vi "ArmR-L-EToXYZ.vi"(9 "Extend":dbl, 10 "Lift":dbl, 11 "Rotate":dbl) -> (1 "z":dbl, 2 "y":dbl, 3 "x":dbl)   [LabVIEW 2020]
uses:
  <vilib>/Rock Robotics/WPI/ThirdParty/JAS_Junk/TrajLib/Trajectory_Library.lvlib
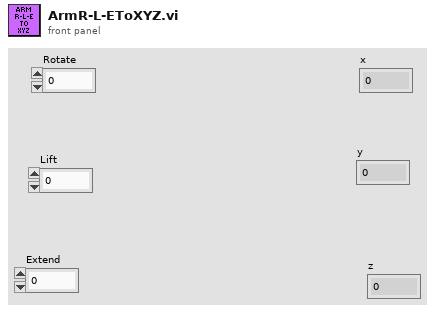
[diagram p1: front panel]
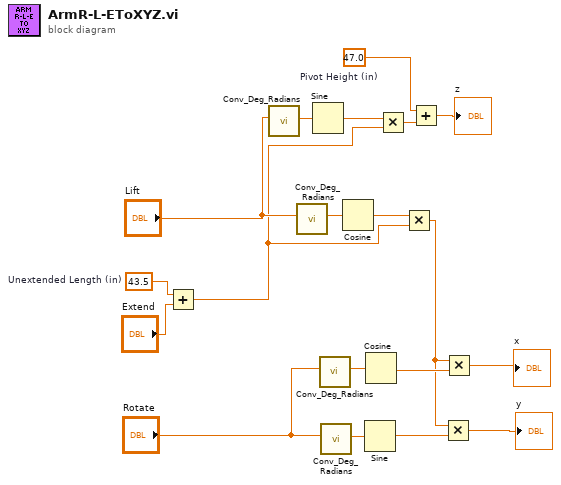
[diagram p0: block diagram]
diagram:
  w1 = 47.0  # Pivot Height (in)
  w18 = 43.5  # Unextended Length (in)
  n1 = Add(x=w18, y="Extend") -> (x+y=w12:dbl)
  n2 = call <vilib>:"Conv_Deg_Radians.vi"("Degress"="Lift") -> ("Radians"=w19:dbl)  [unwired: 10 in]
  n3 = call <vilib>:"Conv_Deg_Radians.vi"("Degress"="Lift") -> ("Radians"=w15:dbl)  [unwired: 10 in]
  n4 = Sine(x=w19) -> (sin(x)=w16:dbl)
  n5 = call <vilib>:"Conv_Deg_Radians.vi"("Degress"="Rotate") -> ("Radians"=w10:dbl)  [unwired: 10 in]
  n6 = call <vilib>:"Conv_Deg_Radians.vi"("Degress"="Rotate") -> ("Radians"=w11:dbl)  [unwired: 10 in]
  n7 = Cosine(x=w15) -> (cos(x)=w13:dbl)
  n8 = Sine(x=w11) -> (sin(x)=w7:dbl)
  n9 = Cosine(x=w10) -> (cos(x)=w6:dbl)
  n10 = Multiply(x=w16, y=w12) -> (x*y=w3:dbl)
  n11 = Multiply(x=w13, y=w12) -> (x*y=w4:dbl)
  n12 = Add(x=w1, y=w3) -> (x+y=→"z":dbl)
  n13 = Multiply(x=w4, y=w7) -> (x*y=→"y":dbl)
  n14 = Multiply(x=w4, y=w6) -> (x*y=→"x":dbl)
